vi "update game parameters.vi"(11 "Difficulty":enum16{"Easy", "Normal", "Hard"}(ring)=enum."Normal") -> (3 "Game Parameters":T1={"Upper Limit (m)"=0.0, "Lower Limit (m)"=0.0, "Obstacle time"=0.0, "Obstacle length"=0.0, "fuel decrement"=0.0, "Fuel time"=0.0, "fuel amount"=0.0, "Fuel range"=0, "Death range"=0, "Terrain slope"=0.0, "Speed (km/hr)"=0.0, "Time step (ms)"=0, "Gravity"=0.0, "Date"="", "High scores path"=path "C:/Users/lz2/Code/LabVIEW/Helicopter/hi scores.txt", "Difficulty"=enum."Normal", "Headstart"=30})   [LabVIEW 2017]
uses:
  controls/game parameters.ctl
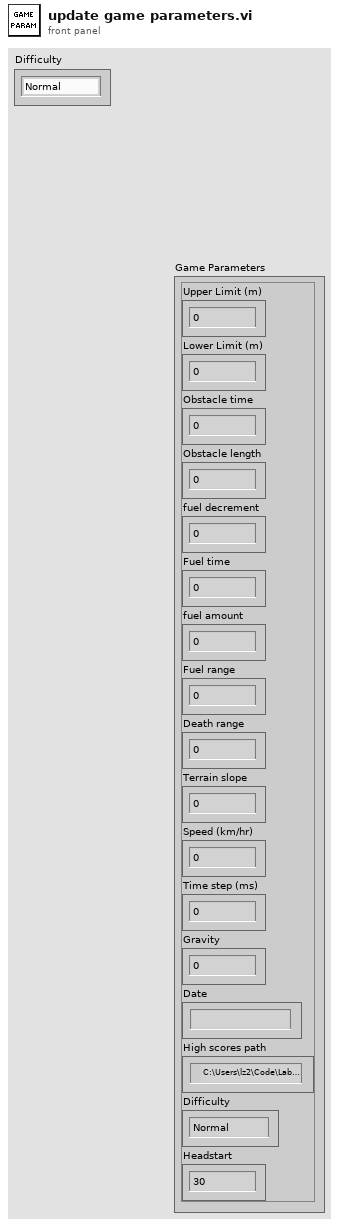
[diagram p1: front panel]
types:
  T1 = typedef "game parameters.ctl" = cluster{"Upper Limit (m)":dbl, "Lower Limit (m)":dbl, "Obstacle time":dbl, "Obstacle length":dbl, "fuel decrement":dbl, "Fuel time":dbl, "fuel amount":dbl, "Fuel range":i32, "Death range":i32, "Terrain slope":dbl, "Speed (km/hr)":dbl, "Time step (ms)":u32, "Gravity":dbl, "Date":string, "High scores path":path, "Difficulty":enum16{"Easy", "Normal", "Hard"}, "Headstart":u32}
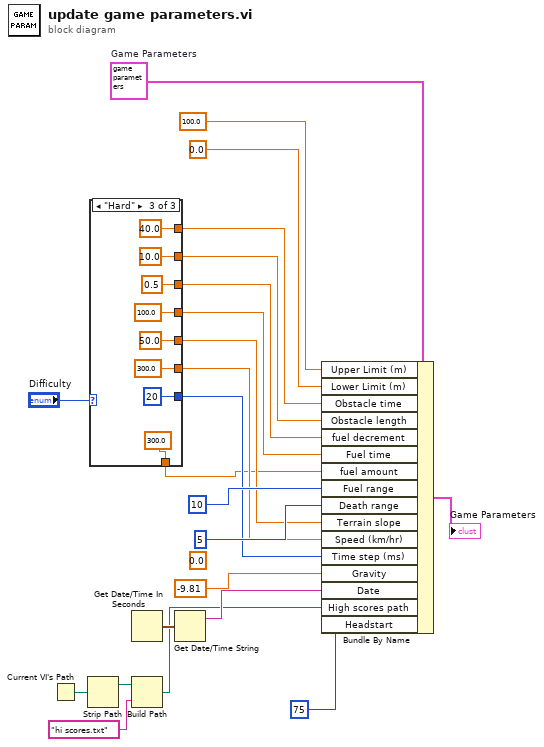
[diagram p0: block diagram]
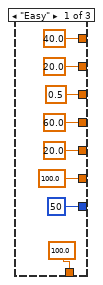
[diagram p2: hidden frame]
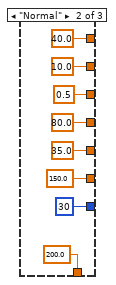
[diagram p3: hidden frame]
diagram:
  (unwired) 0.0 ("Score")
  w22 = T1 {"Upper Limit (m)"=100.0, "Lower Limit (m)"=0.0, "Obstacle time"=20.0, "Obstacle length"=10.0, "fuel decrement"=0.5, "Fuel time"=100.0, "fuel amount"=50.0, "Fuel range"=10, "Death range"=5, "Terrain slope"=35.0, "Speed (km/hr)"=150.0, "Time step (ms)"=30, "Gravity"=-9.81, "Date"="11/03/2016", "High scores path"=path "C:/Users/lz2/Code/LabVIEW/Helicopter/hi scores.txt", "Difficulty"=enum."Normal", "Headstart"=30}  # Game Parameters
  n1 = Current VI's Path() -> (path=w20:path)
  n2 = Strip Path(path=w20) -> (stripped path=w19:path)  [unwired: 1 out]
  n3 = case shown="\"Hard\"" "Difficulty" {
    tunnel: [40.0 ("Obstacle time") 40.0 ("Obstacle time") 40.0 ("Obstacle time")] -> w14
    tunnel: [20.0 ("Terrain slope") 35.0 ("Terrain slope") 50.0 ("Terrain slope")] -> w8
    tunnel: [20.0 ("Obstacle length") 10.0 ("Obstacle length") 10.0 ("Obstacle length")] -> w13
    tunnel: [0.5 ("fuel decrement") 0.5 ("fuel decrement") 0.5 ("fuel decrement")] -> w12
    tunnel: [u32 50 ("Time step (ms)") u32 30 ("Time step (ms)") u32 20 ("Time step (ms)")] -> w6
    tunnel: [60.0 ("fuel decrement") 80.0 ("fuel decrement") 100.0 ("fuel decrement")] -> w11
    tunnel: [100.0 ("Speed (km/hr)") 150.0 ("Speed (km/hr)") 300.0 ("Speed (km/hr)")] -> w7
    tunnel: [100.0 ("fuel amount 2") 200.0 ("fuel amount 2") 300.0 ("fuel amount 2")] -> w1
    frame "Easy" {
    }
    frame "Normal" {
    }
    frame "Hard" {
    }
  }
  n4 = Get Date/Time In Seconds() -> (seconds since 1Jan1904=w21:timestamp)
  n5 = Build Path(base path=w19, name or relative path="hi scores.txt") -> (appended path=w3:path)
  n6 = Get Date/Time String(seconds (now)=w21) -> (date string=w5:string)  [unwired: 2 in, 1 out]
  n7 = Bundle By Name(cluster=w22, "Upper Limit (m)"=100.0, "Lower Limit (m)"=0.0, "Obstacle time"=w14, "Obstacle length"=w13, "fuel decrement"=w12, "Fuel time"=w11, "fuel amount"=w1, "Fuel range"=10 ("Death range"), "Death range"=5, "Terrain slope"=w8, "Speed (km/hr)"=w7, "Time step (ms)"=w6, "Gravity"=-9.81, "Date"=w5, "High scores path"=w3, "Headstart"=u32 75) -> (→"Game Parameters":T1)
